vi "Insert value in Byte.vi"(1 "MSB":u8, 2 "Input (HEX)":u8 format="0x%x", 3 "Value (HEX)":u8 format="0x%x", 4 "LSB":u8) -> (7 "Output (HEX)":u8 format="0x%x")   [LabVIEW 2021]
panel:
  out "output":bool[](array[boolean])
  out "value":bool[](array[boolean])
  out "Input":bool[](array[boolean])
  # "7"
  # "6"
  # "5"
  # "4"
  # "3"
  # "2"
  # "1"
  # "0"
  # "7"
  # "6"
  # "5"
  # "4"
  # "3"
  # "2"
  # "1"
  # "0"
  # "7"
  # "6"
  # "5"
  # "4"
  # "3"
  # "2"
  # "1"
  # "0"
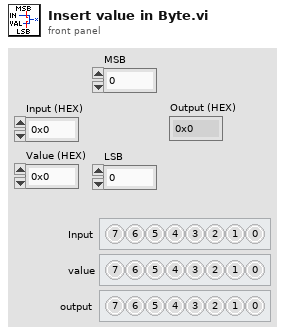
[diagram p1: front panel]
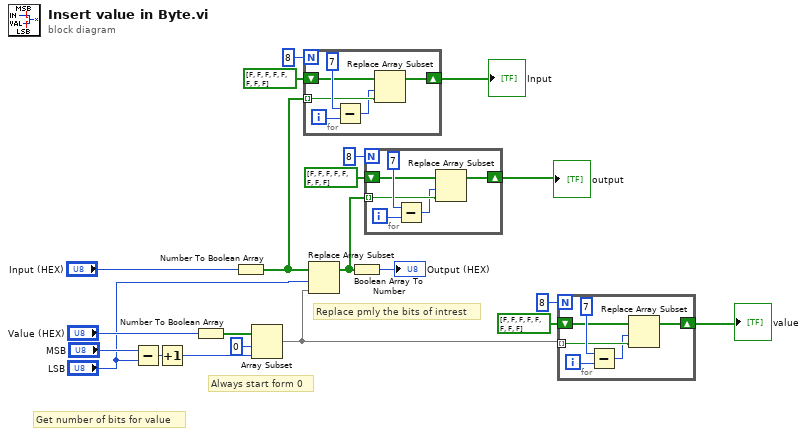
[diagram p0: block diagram]
diagram:
  # "Always start form 0"
  # "Get number of bits for value"
  # "Replace pmly the bits of intrest"
  n1 = Subtract(x="MSB", y="LSB") -> (x-y=w20:u8)
  n2 = Increment(x=w20) -> (x+1=w19:u8)
  n3 = Number To Boolean Array(number="Value (HEX)") -> (Boolean array=w21:bool[])
  n4 = Number To Boolean Array(number="Input (HEX)") -> (Boolean array=w12:bool[])
  n5 = Array Subset(array=w21, index=0, length=w19) -> (w5:bool[])
  n6 = for {
    N: 8 -> [_]
    tunnel: w12 -> [w23] mode=indexing
    shift-right: [w24] -> w2
    shift-left: bool[] [FALSE, FALSE, FALSE, FALSE, FALSE, FALSE, FALSE, FALSE] ("array") -> [w25]
    i -> [w26]
    n7 = Subtract(x=7 ("y"), y=w26) -> (x-y=w22:i32)
    n8 = Replace Array Subset(array=w25, new element=w23, index=w22) -> (w24:bool[])
  }
  "Input" <- w2
  n9 = Replace Array Subset(array=w12, new element=w5, index="LSB") -> (w9:bool[])
  n10 = Boolean Array To Number(Boolean array=w9) -> (number=→"Output (HEX)":u32)
  n11 = for {
    N: 8 -> [_]
    tunnel: w9 -> [w29] mode=indexing
    shift-right: [w30] -> w3
    shift-left: bool[] [FALSE, FALSE, FALSE, FALSE, FALSE, FALSE, FALSE, FALSE] ("array") -> [w31]
    i -> [w32]
    n12 = Subtract(x=7 ("y"), y=w32) -> (x-y=w28:i32)
    n13 = Replace Array Subset(array=w31, new element=w29, index=w28) -> (w30:bool[])
  }
  "output" <- w3
  n14 = for {
    N: 8 -> [_]
    tunnel: w5 -> [w35] mode=indexing
    shift-right: [w36] -> w1
    shift-left: bool[] [FALSE, FALSE, FALSE, FALSE, FALSE, FALSE, FALSE, FALSE] ("array") -> [w37]
    i -> [w38]
    n15 = Subtract(x=7 ("y"), y=w38) -> (x-y=w34:i32)
    n16 = Replace Array Subset(array=w37, new element=w35, index=w34) -> (w36:bool[])
  }
  "value" <- w1
